vi "(10) Move X (Stop and Scan) - Automatic Loop.vi"() -> ()   [LabVIEW 2020]
uses:
  <instrlib>/Arcus Ethernet Driver 1.0.0/ArcusEthernetComm/classes/Controller/_Controller.lvclass
panel:
  in  "Initial Direction":bool
  in  "X Desired Distance (mm)":dbl
  in  "error in (no error)":errorcluster
  in  "Scan":bool
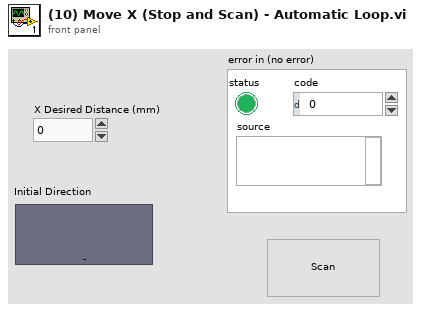
[diagram p1: front panel]
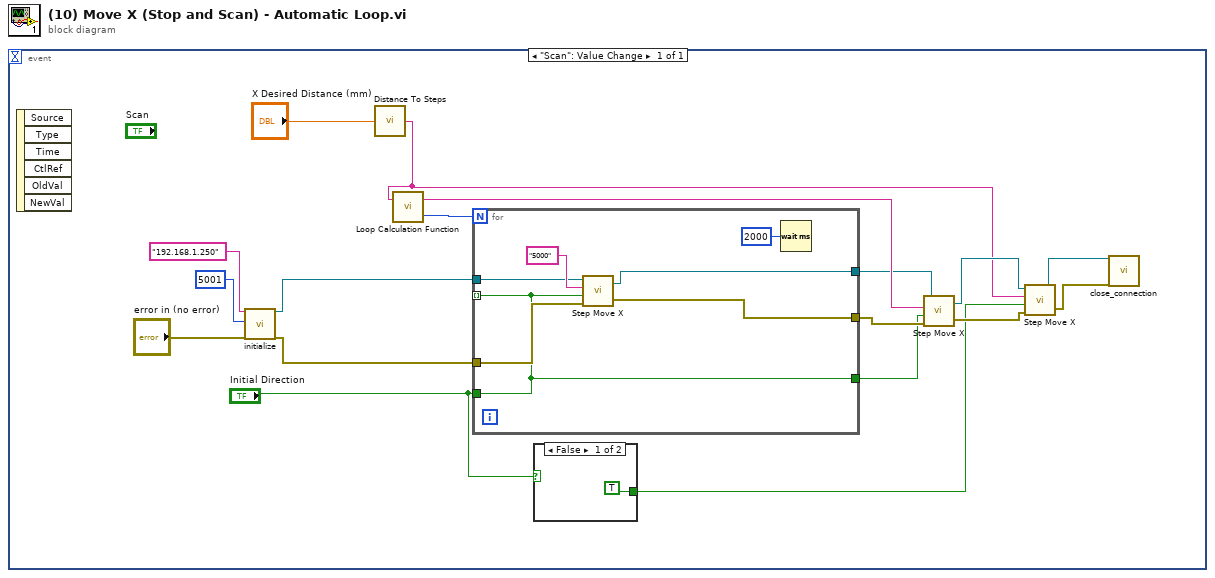
[diagram p0: block diagram]
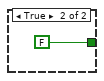
[diagram p2: hidden frame]
diagram:
  n1 = event shown="[0] \"Scan\": Value Change" {
    selector: _ -> [_]
    dyn-events: _ -> [_]
    timeout: _ -> [_]
    event "Scan": Value Change {
      n2 = event-data() -> ()  [unwired: 1 in, 6 out]
      n3 = call <instrlib>:"initialize.vi"("ip_address (in)"="192.168.1.250", "dev_port(def=5001)"=u16 5001, "error in (no error)"="error in (no error)") -> ("reference (out)"=w11:refnum<class "_Controller.lvclass">, "error out"=w12:errorcluster)  [unwired: 15 in]
      n4 = call "Distance To Steps.vi"("Desired Distance (mm)"="X Desired Distance (mm)") -> ("Number of Steps"=w1:string)
      n5 = call "Loop Calculation Function.vi"("Number of Steps"=w1) -> ("No. of Loops (-1)"=w13:i32, "Remainder"=w14:string)  [unwired: 1 in]
      n6 = for {
        N: w13 -> [_]
        tunnel: w12 -> [w25]
        tunnel: [w23] -> w9
        tunnel: [w21] -> _ mode=indexing
        tunnel: "Initial Direction" -> [w21]
        tunnel: w11 -> [w24]
        tunnel: [w22] -> w8
        tunnel: [w21] -> w7
        n7 = call "Step Move X.vi"("error in (no error)"=w25, "Direction"=w21, "x steps"="5000" ("X Steps"), "reference (in)"=w24) -> ("error out"=w22:errorcluster, "reference (out)"=w23:refnum<class "_Controller.lvclass">)
        n8 = Wait (ms)(milliseconds to wait=u32 2000) -> ()  [unwired: 1 out]
      }
      n9 = case shown="False" "Initial Direction" {
        tunnel: [TRUE FALSE] -> w2
        frame False {
        }
        frame True {
        }
      }
      n10 = call "Step Move X.vi"("error in (no error)"=w8, "Direction"=w7, "x steps"=w14, "reference (in)"=w9) -> ("error out"=w3:errorcluster, "reference (out)"=w6:refnum<class "_Controller.lvclass">)
      n11 = call "Step Move X.vi"("error in (no error)"=w3, "Direction"=w2, "x steps"=w1, "reference (in)"=w6) -> ("error out"=w5:errorcluster, "reference (out)"=w4:refnum<class "_Controller.lvclass">)
      n12 = call <instrlib>:"close_connection.vi"("reference (in)"=w4, "error in (no error)"=w5) -> ()  [unwired: 16 in, 2 out]
    }
  }
